vi "LOT_Select_Wavelength.vi"(0 "Input Wavelength":dbl) -> (1 "Error Code":i32, 2 "Current Wavelength":dbl)   [LabVIEW 2023]
uses:
  SN19523/LOThw/LOThw64.dll
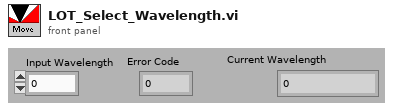
[diagram p1: front panel]
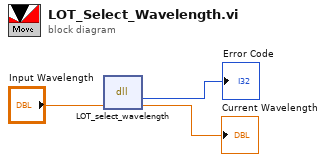
[diagram p0: block diagram]
diagram:
  n1 = dll-call lib="E:/Old PC/desktop/Sensitive EQE Stuff/S-EQE (YJ)/LOT/SN19523/LOThw/LOThw64.dll" fn="LOT_select_wavelength"("wl"="Input Wavelength") -> ("return type"=→"Error Code":i16, "wl"=→"Current Wavelength":dbl)  [unwired: 3 in, 2 out]
